vi "New TipTable.vi"(7 "show.color":T1, 8 "error in (no error)":errorcluster, 9 "show.Column Headers":string[](array[string]), 10 "show.Row Headers":string[](array[string]), 11 "show.cells":T2[][](array[typedef])) -> (0 "error out":errorcluster, 3 "TipTablePanel out":refnum<class "TipTablePanel.lvclass">)   [LabVIEW 2021, in "RocketPlot.lvlib" / "TipTablePanel.lvclass"]
uses:
  TipTablePanel.lvclass
  cell cache.ctl
  colors.ctl
  TipTablePanel.lvclass/TipTablePanel.ctl
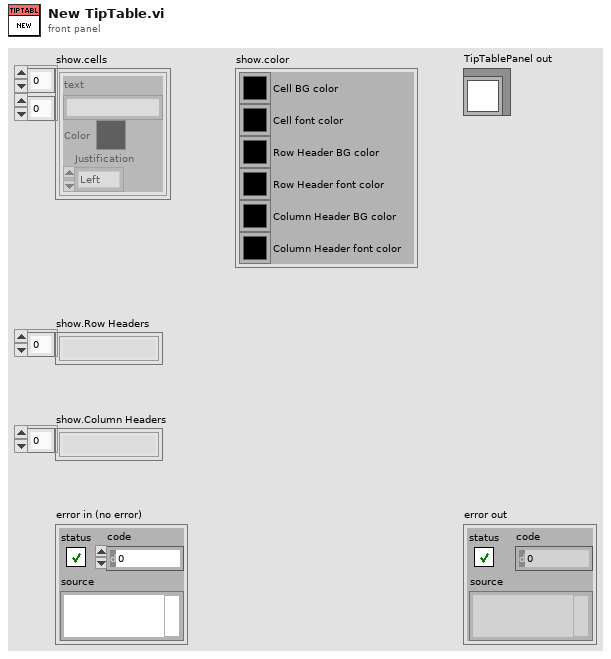
[diagram p1: front panel]
types:
  T1 = typedef "RocketPlot.lvlib/TipTablePanel.lvclass/colors.ctl" = cluster{"Cell BG color":u32, "Cell font color":u32, "Row Header BG color":u32, "Row Header font color":u32, "Column Header BG color":u32, "Column Header font color":u32}
  T2 = typedef "RocketPlot.lvlib/TipTablePanel.lvclass/cell cache.ctl" = cluster{"text":string, "Color":u32, "Justification":enum16{"Left", "Center", "Right"}}
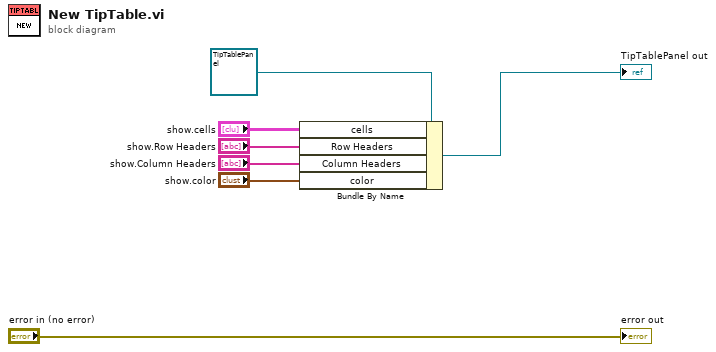
[diagram p0: block diagram]
diagram:
  n1 = Bundle By Name(cluster=refnum<class "TipTablePanel.lvclass"> refnum ("TipTablePanel out"), "cells"="show.cells", "Row Headers"="show.Row Headers", "Column Headers"="show.Column Headers", "color"="show.color") -> (→"TipTablePanel out":refnum<class "TipTablePanel.lvclass">)
  "error out" <- "error in (no error)"
